vi "DesiredLevelStateMachine.vi"   [LabVIEW 2014]
uses:
  DesiredLevelStates.ctl
  Global Data!!!.vi
types:
  T1 = typedef "DesiredLevelStates.ctl" = enum16{"No Change", "Change"}
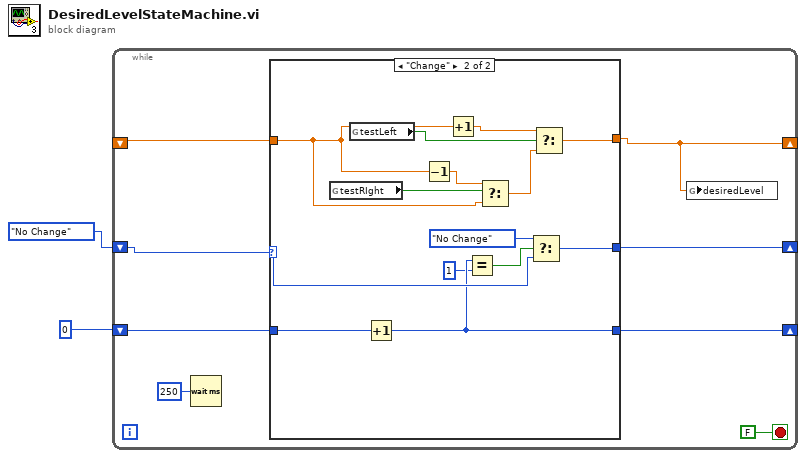
[diagram p0: block diagram]
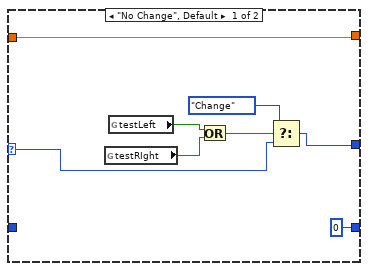
[diagram p2: hidden frame]
diagram:
  n1 = while {
    shift-right: [w7] -> _
    shift-left: DesiredLevelStates."No Change" -> [w10]
    shift-right: [w8] -> _
    shift-left: _ -> [w9]
    shift-right: [w5] -> _
    shift-left: 0 -> [w6]
    stop <- FALSE stop-if-true
    n2 = Wait (ms)(milliseconds to wait=u32 250) -> ()  [unwired: 1 out]
    n3 = case shown="\"Change\"" w10 {
      selector: w10 -> [w14 w25]
      tunnel: [w18 w29] -> w8
      tunnel: w9 -> [w18 w19]
      tunnel: [w13 w26] -> w7
      tunnel: w6 -> [_ w23]
      tunnel: [0 w21] -> w5
      frame "No Change", Default {
        n4 = global read "Global Data!!!.vi" "testRIght"() -> (w16:bool)
        n5 = global read "Global Data!!!.vi" "testLeft"() -> (w17:bool)
        n6 = Or(x=w17, y=w16) -> (x .or. y?=w15:bool)
        n7 = Select(t=DesiredLevelStates."Change", s=w15, f=w14) -> (s? t:f=w13:T1)
      }
      frame "Change" {
        n8 = global read "Global Data!!!.vi" "testRIght"() -> (w30:bool)
        n9 = global read "Global Data!!!.vi" "testLeft"() -> (w31:bool)
        n10 = Increment(x=w23) -> (x+1=w21:i32)
        n11 = Decrement(x=w19) -> (x-1=w28:dbl)
        n12 = Increment(x=w19) -> (x+1=w27:dbl)
        n13 = Equal?(x=w21, y=1) -> (x = y?=w22:bool)
        n14 = Select(t=w28, s=w30, f=w19) -> (s? t:f=w32:dbl)
        n15 = Select(t=DesiredLevelStates."No Change", s=w22, f=w25) -> (s? t:f=w26:T1)
        n16 = Select(t=w27, s=w31, f=w32) -> (s? t:f=w29:dbl)
      }
    }
    n17 = global write "Global Data!!!.vi" "desiredLevel"(w8) -> ()
  }
